vi "Timeout.vi"(8 "error in":errorcluster, 11 "Modbus master in":refnum<class "Modbus Master.lvclass">) -> (0 "error out":errorcluster, 1 "Boolean":bool, 3 "Modbus master out":refnum<class "Modbus Master.lvclass">, 9 "Timer":u16, 10 "Temperature":u16)   [LabVIEW 2014, in "Main Libraryv2.lvlib"]
uses:
  Control/Main Libraryv2.lvlib
  <vilib>/NI/Modbus Library/API/Master/Modbus Master.lvclass
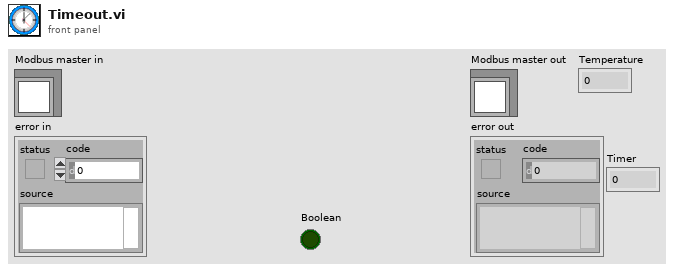
[diagram p1: front panel]
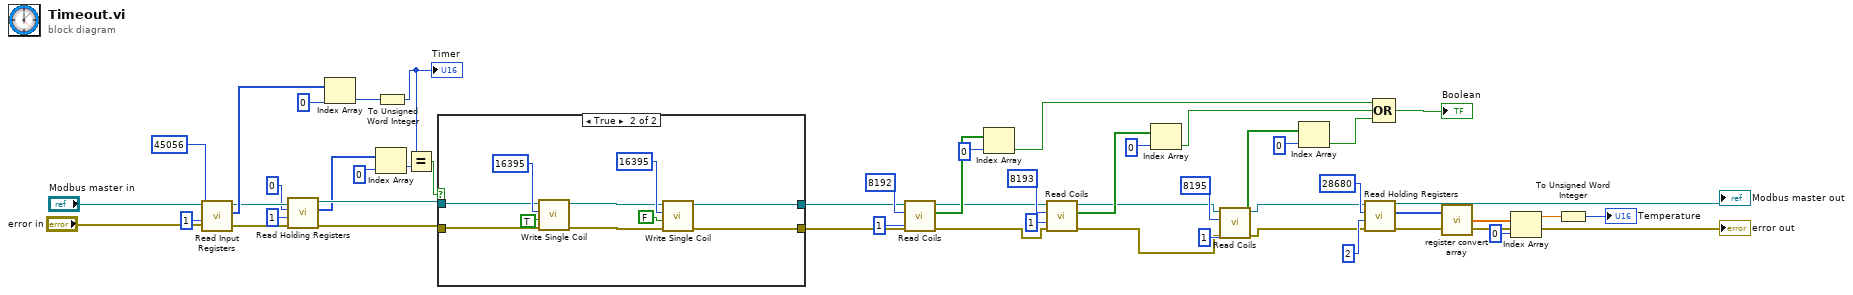
[diagram p0: block diagram]
diagram:
  n1 = call-dynamic "Read Input Registers.vi"("error in"="error in", "number of inputs"=u16 1, "starting address"=u16 45056, "Modbus master in"="Modbus master in") -> ("error out"=w30:errorcluster, "register values"=w36:u16[], "Modbus master out"=w33:refnum<class "Modbus Master.lvclass">)  [unwired: 5 in]
  n2 = call-dynamic "Read Holding Registers.vi"("error in"=w30, "number of inputs"=u16 1, "starting address"=u16 0, "Modbus master in"=w33) -> ("error out"=w31:errorcluster, "register values"=w27:u16[], "Modbus master out"=w32:refnum<class "Modbus Master.lvclass">)  [unwired: 5 in]
  n3 = Index Array(array=w36, index=0) -> (element=w37:u16)
  n4 = Index Array(array=w27, index=0) -> (element=w25:u16)
  n5 = To Unsigned Word Integer(number=w37) -> (unsigned 16bit integer=w34:u16)
  "Timer" <- w34
  n6 = Equal?(x=w34, y=w25) -> (x = y?=w35:bool)
  n7 = case shown="True" w35 {
    tunnel: w32 -> [w53 w57]
    tunnel: w31 -> [w52 w56]
    tunnel: [w53 w55] -> w12
    tunnel: [w52 w54] -> w11
    frame False {
    }
    frame True {
      n8 = call-dynamic "Write Single Coil.vi"("error in"=w56, "coil to write"=TRUE, "address"=u16 16395, "Modbus master in"=w57) -> ("error out"=w61:errorcluster, "Modbus master out"=w60:refnum<class "Modbus Master.lvclass">)  [unwired: 6 in]
      n9 = call-dynamic "Write Single Coil.vi"("error in"=w61, "coil to write"=FALSE, "address"=u16 16395, "Modbus master in"=w60) -> ("error out"=w54:errorcluster, "Modbus master out"=w55:refnum<class "Modbus Master.lvclass">)  [unwired: 6 in]
    }
  }
  n10 = call-dynamic "Read Coils.vi"("error in"=w11, "number of inputs"=u16 1, "starting address"=u16 8192, "Modbus master in"=w12) -> ("error out"=w10:errorcluster, "coils"=w22:bool[], "Modbus master out"=w9:refnum<class "Modbus Master.lvclass">)  [unwired: 5 in]
  n11 = Index Array(array=w22, index=0) -> (element=w4:bool)
  n12 = call-dynamic "Read Coils.vi"("error in"=w10, "number of inputs"=u16 1, "starting address"=u16 8193, "Modbus master in"=w9) -> ("error out"=w7:errorcluster, "coils"=w18:bool[], "Modbus master out"=w8:refnum<class "Modbus Master.lvclass">)  [unwired: 5 in]
  n13 = Index Array(array=w18, index=0) -> (element=w3:bool)
  n14 = call-dynamic "Read Coils.vi"("error in"=w7, "number of inputs"=u16 1, "starting address"=u16 8195, "Modbus master in"=w8) -> ("error out"=w5:errorcluster, "coils"=w14:bool[], "Modbus master out"=w6:refnum<class "Modbus Master.lvclass">)  [unwired: 5 in]
  n15 = Index Array(array=w14, index=0) -> (element=w2:bool)
  n16 = call-dynamic "Read Holding Registers.vi"("error in"=w5, "number of inputs"=u16 2, "starting address"=u16 28680, "Modbus master in"=w6) -> ("error out"=→"error out":errorcluster, "register values"=w43:u16[], "Modbus master out"=→"Modbus master out":refnum<class "Modbus Master.lvclass">)  [unwired: 5 in]
  n17 = Compound Arithmetic op=OR(w4, w3, w2) -> (→"Boolean":bool)
  n18 = call "register convert array.vi"("Register Array"=w43) -> ("Converted Array"=w41:sgl[])  [unwired: 1 in]
  n19 = Index Array(array=w41, index=0) -> (element=w39:sgl)
  n20 = To Unsigned Word Integer(number=w39) -> (unsigned 16bit integer=→"Temperature":u16)
